vi "RS-xxx to GPIB ConvBox Factory.vi"(8 "error in":errorcluster, 10 "RS-xxx to GPIB ConvBox settings":T1) -> (0 "error out":errorcluster, 3 "RS-xxx to GPIB ConvBox Out":refnum<class "RS-xxx to GPIB ConvBox.lvclass">)   [LabVIEW 2018, in "Protocols.lvlib" / "RS-xxx to GPIB ConvBox.lvclass"]
doc: "Instantiates an RS-xxx to GPIB ConvBox object using the provided RS-xxx to GPIB ConvBox Settings"
uses:
  RS-xxx to GPIB ConvBox.lvclass
  RS-xxx to GPIB ConvBox Settings.ctl
  RS-xxx to GPIB ConvBox.lvclass/RS-xxx to GPIB ConvBox.ctl
  Data Access/Write Port.vi
  Data Access/Write ConvBox Address.vi
  Data Access/Write Assert Ren with IFC.vi
  Data Access/Write System controller.vi
  Data Access/Write IST bit sense.vi
  Data Access/Write GPIB Address.vi
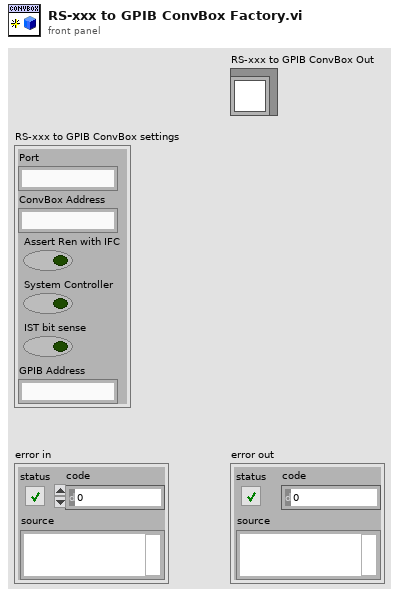
[diagram p1: front panel]
types:
  T1 = typedef "Protocols.lvlib/RS-xxx to GPIB ConvBox.lvclass/RS-xxx to GPIB ConvBox Settings.ctl" = cluster{"Port":string, "ConvBox Address":string, "Assert Ren with IFC":bool, "System Controller":bool, "IST bit sense":bool, "GPIB Address":string}
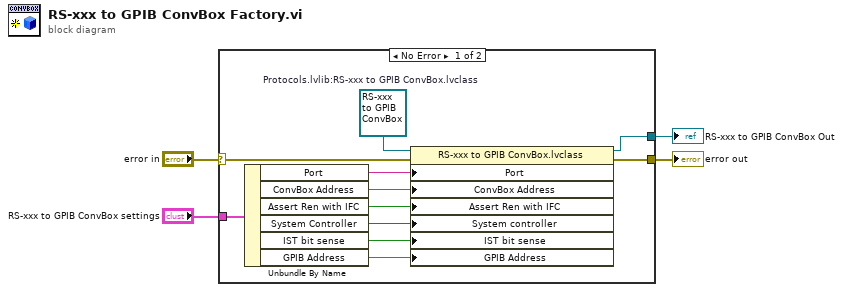
[diagram p0: block diagram]
diagram:
  n1 = case shown="No Error" "error in" {
    selector: "error in" -> [w5 w16]
    tunnel: "RS-xxx to GPIB ConvBox settings" -> [w15 _]
    tunnel: [w13 _] -> w3
    tunnel: [w12 w16] -> w2
    frame No Error {
      w14 = refnum<class "RS-xxx to GPIB ConvBox.lvclass"> refnum  # Protocols.lvlib:RS-xxx to GPIB ConvBox.lvclass
      n2 = Unbundle By Name(w15) -> ("Port"=w11:string, "ConvBox Address"=w10:string, "Assert Ren with IFC"=w9:bool, "System Controller"=w8:bool, "IST bit sense"=w7:bool, "GPIB Address"=w6:string)
      n3 = property class="RS-xxx to GPIB ConvBox.lvclass"(reference=w14, error in=w5, "Port"=w11, "ConvBox Address"=w10, "Assert Ren with IFC"=w9, "System controller"=w8, "IST bit sense"=w7, "GPIB Address"=w6) -> (reference out=w13:refnum<class "RS-xxx to GPIB ConvBox.lvclass">, error out=w12:errorcluster)
    }
    frame Error {
    }
  }
  "RS-xxx to GPIB ConvBox Out" <- w3
  "error out" <- w2
